vi "Msg Rescript.vi"() -> ()   [LabVIEW 2021]
uses:
  _Shared/_Shared.lvlib
  _Msg Rescript/_Msg Rescript/_Msg Rescript.lvclass
panel:
  in  "Rescript":bool
  in  "Name":string(combo)
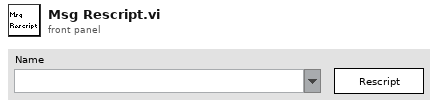
[diagram p1: front panel]
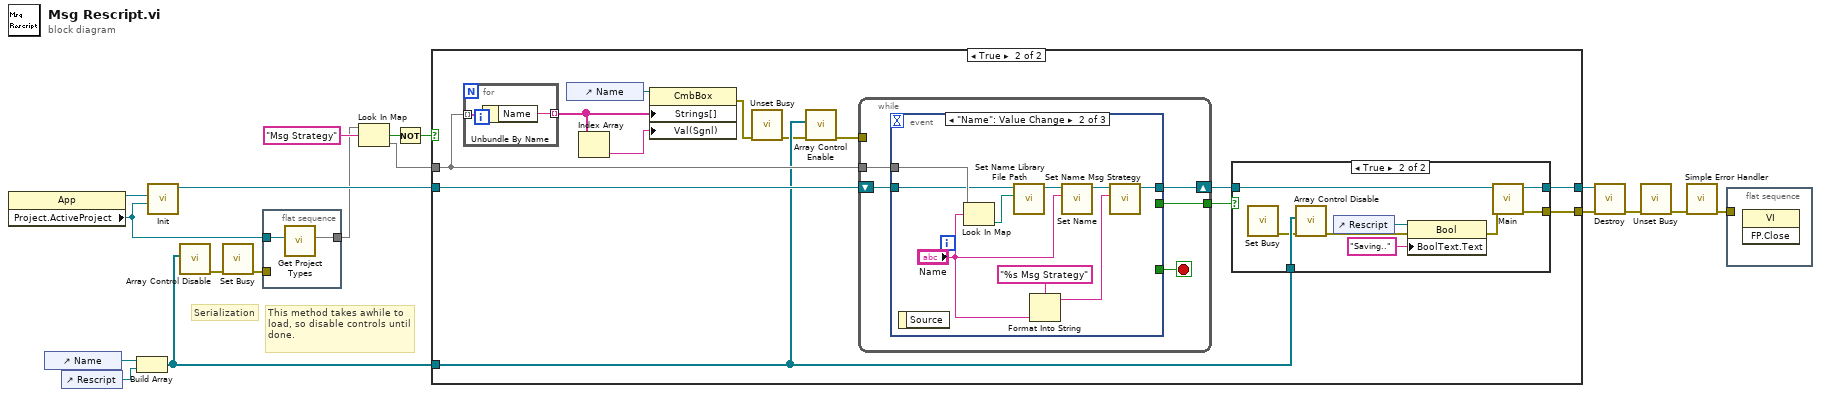
[diagram p0: block diagram]
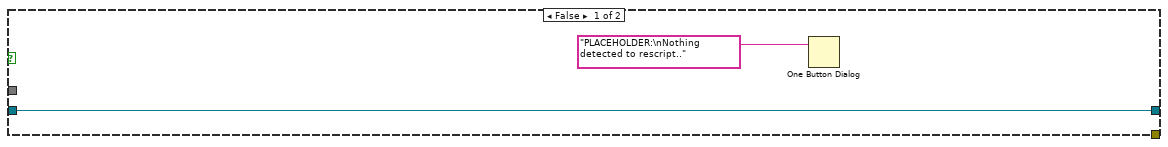
[diagram p2: hidden frame]
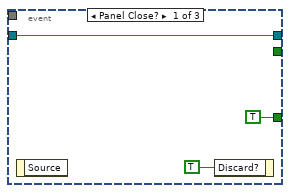
[diagram p4: hidden frame]
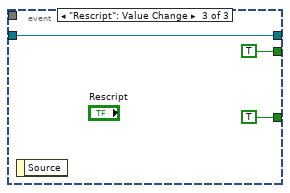
[diagram p5: hidden frame]
diagram:
  # "Serialization"
  # "This method takes awhile to load, so disable controls until done."
  n1 = property class="App"() -> (reference out=w13:refnum<vi>, "Project.ActiveProject"=w12:refnum<vi>)  [unwired: 2 in, 1 out]
  n2 = control-ref of="Name"() -> (w10:refnum<vi>)
  n3 = control-ref of="Rescript"() -> (w9:refnum<vi>)
  n4 = Build Array(w10, w9) -> (w18:refnum<vi>[])
  n5 = call "Init.vi"("Project:Active Project"=w12, "NI.LV.Dialog Instance"=w13) -> ("_Rescript Msg out"=w11:refnum<class "_Msg Rescript.lvclass">)  [unwired: 8 in, 1 out]
  n6 = call "Array Control Disable.vi"("Array Control in"=w18) -> ("error out"=w16:errorcluster)  [unwired: 10 in]
  n7 = call <vilib>:"Set Busy.vi"("error in (no error)"=w16) -> ("error out"=w15:errorcluster)  [unwired: 9 in, 1 out]
  n8 = flat-sequence {
    tunnel: w12 -> [w20]
    tunnel: [w19] -> w4
    tunnel: w15 -> [_]
    frame #0 {
      n9 = call "Get Project Types.vi"("Project:Active Project"=w20) -> ("Type Name Library File Path"=w19:map{string, map{string, path}})  [unwired: 10 in]
    }
  }
  n10 = Look In Map(map=w4, key="Msg Strategy" ("y")) -> (key not found?=w2:bool, value=w3:map{string, path})  [unwired: 1 in]
  n11 = Not(x=w2) -> (.not. x?=w1:bool)
  n12 = case shown="True" w1 {
    tunnel: w11 -> [w21 w32]
    tunnel: w3 -> [_ w28]
    tunnel: w18 -> [_ w25]
    tunnel: [w21 w31] -> w8
    tunnel: [_ w30] -> w7
    frame False {
      n13 = One Button Dialog(message="PLACEHOLDER:\nNothing detected to rescript..") -> ()  [unwired: 1 in, 1 out]
    }
    frame True {
      n14 = for {
        tunnel: w28 -> [w37] mode=indexing
        tunnel: [w36] -> w27 mode=indexing
        n15 = Unbundle By Name(w37) -> ("Name"=w36:string)
      }
      n16 = control-ref of="Name"() -> (w26:refnum<vi>)
      n17 = Index Array(array=w27) -> (element=w34:string)  [unwired: 1 in]
      n18 = property class="CmbBox"(reference=w26, "Strings[]"=w27, "Val(Sgnl)"=w34) -> (error out=w29:errorcluster)  [unwired: 1 in, 1 out]
      n19 = call <vilib>:"Unset Busy.vi"("error in (no error)"=w29) -> ("error out"=w24:errorcluster)  [unwired: 10 in]
      n20 = call "Array Control Enable.vi"("error in"=w24, "Array Control in"=w25) -> ("error out"=w23:errorcluster)  [unwired: 9 in]
      n21 = while {
        tunnel: [w52] -> w35
        shift-right: [w49] -> w33
        shift-left: w32 -> [w50]
        tunnel: w28 -> [w48]
        tunnel: w23 -> [_]
        stop <- w51 stop-if-true
        n22 = event shown="[1] \"Name\": Value Change" {
          selector: _ -> [_ _ _]
          dyn-events: _ -> [_ _ _]
          timeout: _ -> [_ _ _]
          tunnel: [_ _ TRUE ("Rename 2")] -> w52
          tunnel: [TRUE _ TRUE] -> w51
          tunnel: w50 -> [w53 w62 w67]
          tunnel: [w53 w59 w67] -> w49
          tunnel: w48 -> [_ w64 _]
          event Panel Close? {
            n23 = event-data() -> ()  [unwired: 1 in, 1 out]
            n24 = event-data("Discard?"=TRUE) -> ()  [unwired: 1 in, 1 out]
          }
          event "Name": Value Change {
            n25 = event-data() -> ()  [unwired: 1 in, 1 out]
            n26 = Look In Map(map=w64, key="Name") -> (value=w63:path)  [unwired: 1 in, 1 out]
            n27 = call "Set Name Library File Path.vi"("Name Library File Path"=w63, "_Rescript Msg in"=w62) -> ("_Rescript Msg out"=w60:refnum<class "_Msg Rescript.lvclass">)  [unwired: 9 in]
            n28 = Format Into String(format string="%s Msg Strategy", "Name") -> (resulting string=w57:string)  [unwired: 2 in, 1 out]
            n29 = call "Set Name.vi"("Name"="Name", "_Rescript Msg in"=w60) -> ("_Rescript Msg out"=w61:refnum<class "_Msg Rescript.lvclass">)  [unwired: 9 in]
            n30 = call "Set Name Msg Strategy.vi"("Name Msg Strategy"=w57, "_Rescript Msg in"=w61) -> ("_Rescript Msg out"=w59:refnum<class "_Msg Rescript.lvclass">)  [unwired: 9 in]
          }
          event "Rescript": Value Change {
            n31 = event-data() -> ()  [unwired: 1 in, 1 out]
          }
        }
      }
      n32 = case shown="True" w35 {
        tunnel: w33 -> [w38 w43]
        tunnel: [w38 w42] -> w31
        tunnel: w25 -> [_ w45]
        tunnel: [_ w40] -> w30
        frame False {
        }
        frame True {
          n33 = call <vilib>:"Set Busy.vi"() -> ("error out"=w44:errorcluster)  [unwired: 10 in, 1 out]
          n34 = call "Array Control Disable.vi"("error in"=w44, "Array Control in"=w45) -> ("error out"=w47:errorcluster)  [unwired: 9 in]
          n35 = control-ref of="Rescript"() -> (w39:refnum<vi>)
          n36 = property class="Bool"(reference=w39, error in=w47, "BoolText.Text"="Saving.." ("Boolean Text.Text")) -> (error out=w41:errorcluster)  [unwired: 1 out]
          n37 = call "Main.vi"("error in"=w41, "_Rescript Msg in"=w43) -> ("error out"=w40:errorcluster, "_Rescript Msg out"=w42:refnum<class "_Msg Rescript.lvclass">)  [unwired: 8 in]
        }
      }
    }
  }
  n38 = call "Destroy.vi"("error in"=w7, "_Rescript Msg in"=w8) -> ("error out"=w6:errorcluster)  [unwired: 9 in]
  n39 = call <vilib>:"Unset Busy.vi"("error in (no error)"=w6) -> ("error out"=w14:errorcluster)  [unwired: 10 in]
  n40 = call <vilib>:"Simple Error Handler.vi"("error in (no error)"=w14) -> ("error out"=w17:errorcluster)  [unwired: 4 in, 4 out]
  n41 = flat-sequence {
    tunnel: w17 -> [_]
    frame #0 {
      n42 = invoke class="VI" method="FP.Close"() -> ()  [unwired: 3 in, 3 out]
    }
  }
